vi "Create Reader Endpoint.vi"(8 "error in (no error)":errorcluster, 9 "writer name":string, 10 "reader name":string, 11 "Stream in":refnum<class "Stream.lvclass">) -> (0 "error out":errorcluster, 3 "Stream out":refnum<class "Stream.lvclass">)   [LabVIEW 2018, in "Stream.lvclass"]
doc: "Create reader endpoint"
uses:
  Stream.lvclass
  Stream.lvclass/Stream.ctl
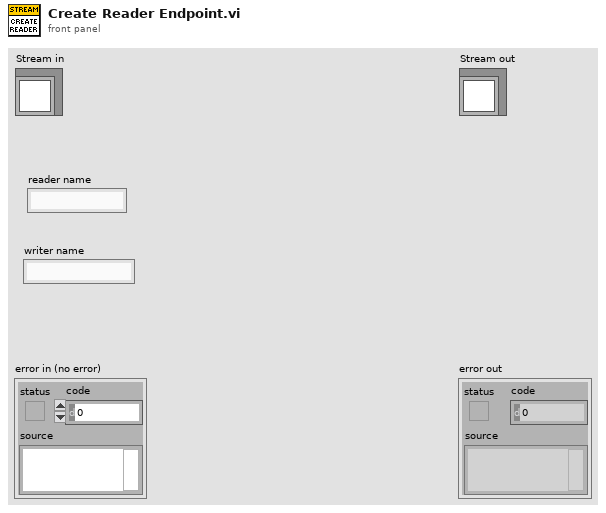
[diagram p1: front panel]
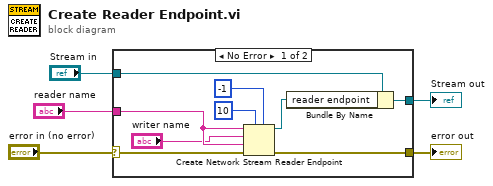
[diagram p0: block diagram]
diagram:
  n1 = case shown="No Error" "error in (no error)" {
    selector: "error in (no error)" -> [w13 w16]
    tunnel: [w14 w16] -> w3
    tunnel: [w10 w15] -> w2
    tunnel: "Stream in" -> [w11 w15]
    tunnel: "reader name" -> [w8 _]
    frame No Error {
      n2 = Create Network Stream Reader Endpoint(5:-1 ("timeout in ms (-1)"), 7:10 ("writer buffer size"), 8:w13, 9:w8, 10:"writer name", 11:w8) -> (0:w14:errorcluster, 3:w7:refnum<k21>)  [unwired: 1 in]
      n3 = Bundle By Name(cluster=w11, "reader endpoint"=w7) -> (w10:refnum<class "Stream.lvclass">)
    }
    frame Error {
    }
  }
  "error out" <- w3
  "Stream out" <- w2
